vi "IsVIInvilib.vi"(11 "ProjectItem in":refnum<vi>) -> (2 "Part of vi.lib?":bool, 3 "ProjectItem out":refnum<vi>)   [LabVIEW 2016, in "NI_NPW_Project Copying.lvlib"]
uses:
  <resource>/dialog/NewProjectWizard/Project Copying/NI_NPW_Project Copying.lvlib
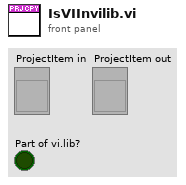
[diagram p1: front panel]
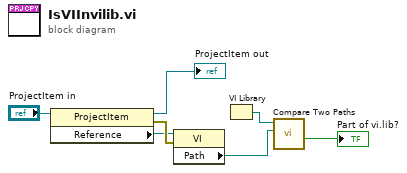
[diagram p0: block diagram]
diagram:
  n1 = property class="ProjectItem"(reference="ProjectItem in") -> (reference out=→"ProjectItem out":refnum<vi>, error out=w6:errorcluster, "Reference"=w5:refnum<vi>)  [unwired: 1 in]
  n2 = property class="VI"(reference=w5, error in=w6) -> ("Path"=w2:path)  [unwired: 2 out]
  n3 = VI Library() -> (path=w3:path)
  n4 = call <vilib>:"Compare Two Paths.vi"("Path 2"=w2, "Path 1"=w3) -> ("Path 2 Relative to Path 1?"=→"Part of vi.lib?":bool)  [unwired: 6 in, 3 out]
